vi "2100_Bridge_Read_Multiple_Registers.vi"(7 "USID":T2 max=15, 8 "Error In":errorcluster, 9 "Reg_Address_to_Read":T4={"First Reg Address"=31, "Num of Reg to Read"=1} {"Num of Reg to Read" min=1; "First Reg Address" format="%.0x"}, 10 "Pins":string[](array[string])=["CLK", "SDA"], 11 "Semiconductor Module Context":T3) -> (0 "Error Out":errorcluster, 2 "Reg_Data":u8[](array[numeric]), 3 "Readback_Array":T1[](array[typedef]) {"Address" format="%.0x"})   [LabVIEW 2013]
uses:
  <vilib>/NI_TestStand_SemiconductorModule/NI_TestStand_Semiconductor_Module.lvlibp/PinMap/General/SemiconductorModuleContext.ctl
  Controls/USID.ctl
  Controls/Reg_Address_Data.ctl
  <vilib>/NI_TestStand_SemiconductorModule/NI_TestStand_Semiconductor_Module.lvlibp
panel:
  out "Converted Data":T5 {"Register" max=31 format="%.0x"; "Slave Address" max=15 format="%.0x"}
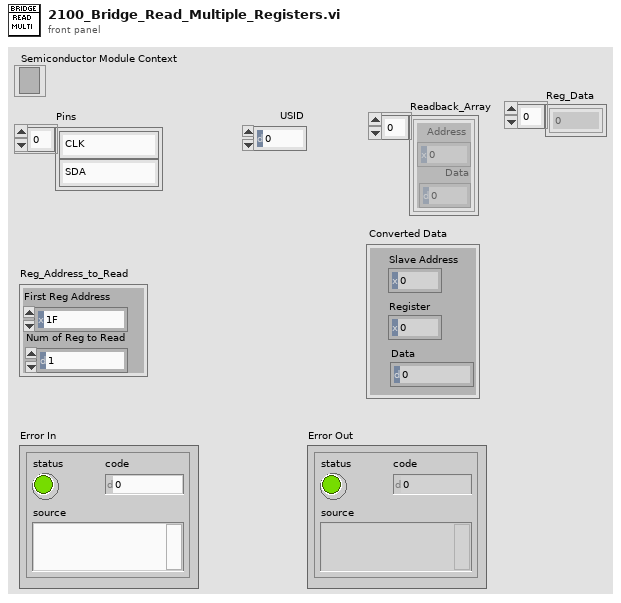
[diagram p1: front panel]
types:
  T1 = typedef "Reg_Address_Data.ctl" = cluster{"Address":u8, "Data":u8}
  T2 = typedef "USID.ctl" = u8
  T3 = typedef "NI_TestStand_Semiconductor_Module.lvlibp/SemiconductorModuleContext.ctl" = refnum<k7>
  T4 = cluster{"First Reg Address":u8, "Num of Reg to Read":u8}
  T5 = cluster{"Slave Address":u8, "Register":u8, "Data":u8}
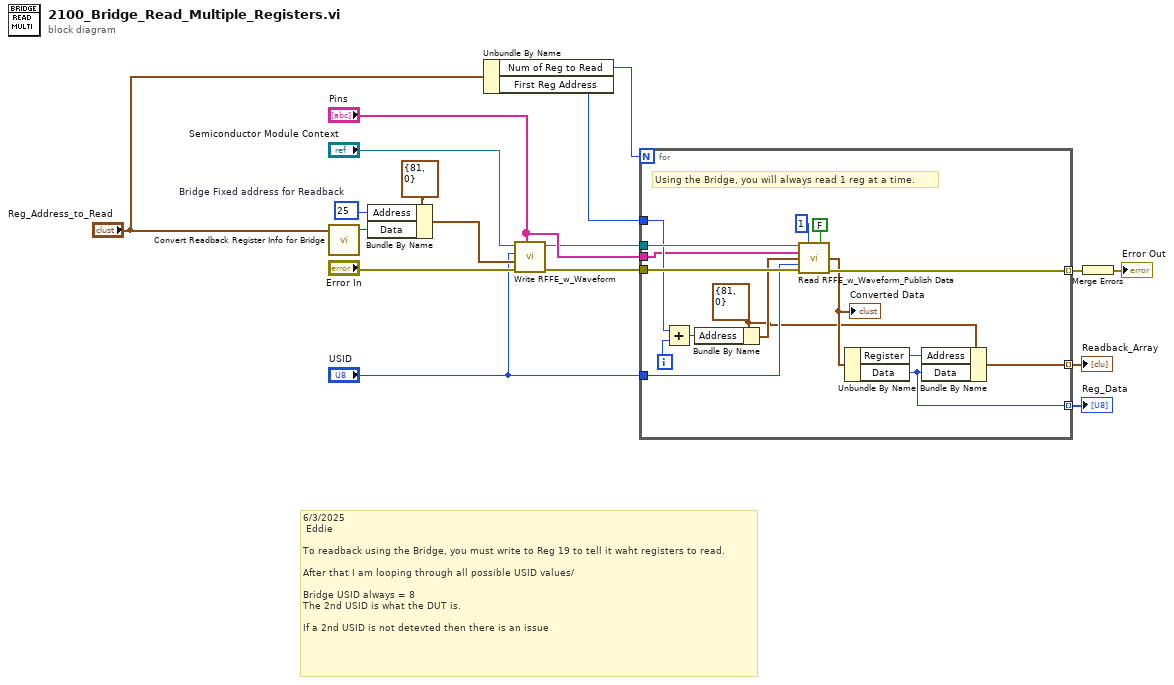
[diagram p0: block diagram]
diagram:
  w15 = u8 25  # Bridge Fixed address for Readback
  # "6/3/2025\n Eddie\n\nTo readback using the Bridge, you must write to Reg 19 to tell it waht registers to read.\n\nAfter that I am looping through all possible USID values/ \n\nBridge USID always = 8\nThe 2nd USID is what the DUT is.\n\nIf a 2nd USID is not detevted then there is an issue"
  n1 = call "Convert Readback Register Info for Bridge.vi"("Reg_Address_to_Read"="Reg_Address_to_Read") -> ("number"=w16:u32)  [unwired: 4 in]
  n2 = Bundle By Name(cluster=T1 {"Address"=81, "Data"=0} ("Reg_Address_Data"), "Address"=w15, "Data"=w16) -> (w13:T1)
  n3 = Unbundle By Name("Reg_Address_to_Read") -> ("Num of Reg to Read"=w4:u8, "First Reg Address"=w7:u8)
  n4 = call "Write RFFE_w_Waveform.vi"("Pins"="Pins", "error in (no error)"="Error In", "Reg_Address_Data"=w13, "USID"="USID", "Semiconductor Module Context"="Semiconductor Module Context") -> ("error out"=w5:errorcluster, "Semiconductor Module Context Out"=w6:T3)  [unwired: 5 in]
  n5 = for {
    N: w4 -> [_]
    tunnel: w7 -> [w26]
    tunnel: w6 -> [w29]
    tunnel: w5 -> [w28]
    tunnel: "Pins" -> [w25]
    tunnel: [w24] -> w10 mode=indexing
    tunnel: "USID" -> [w23]
    tunnel: [w19] -> w2 mode=indexing
    tunnel: [w18] -> w1 mode=indexing
    i -> [w33]
    w21 = T1 {"Address"=81, "Data"=0} ("Reg_Address_Data")
    # "Using the Bridge, you will always read 1 reg at a time."
    n6 = Add(x=w26, y=w33) -> (x+y=w32:i32)
    n7 = Bundle By Name(cluster=w21, "Address"=w32) -> (w27:T1)
    n8 = call "Read RFFE_w_Waveform_Publish Data.vi"("Semiconductor Module Context"=w29, "Num_Reg_to_Read"=u8 1, "Publish_Data?"=FALSE, "Pins"=w25, "Reg_Address_Data"=w27, "USID"=w23, "Error In"=w28) -> ("Converted Data"=w22:T5, "Error Out"=w24:errorcluster)  [unwired: 4 in, 3 out]
    "Converted Data" <- w22
    n9 = Unbundle By Name(w22) -> ("Register"=w20:u8, "Data"=w18:u8)
    n10 = Bundle By Name(cluster=w21, "Address"=w20, "Data"=w18) -> (w19:T1)
  }
  "Readback_Array" <- w2
  "Reg_Data" <- w1
  n11 = Merge Errors(w10) -> (→"Error Out":errorcluster)
